vi "GetHeader2.vi"(8 "error in (no error)":errorcluster caption="에러 입력(에러 없음)", 11 "ABF1FIO 입력":refnum<class "ABF1FIO.lvclass">) -> (0 "error out":errorcluster caption="에러 출력", 1 "Header":T1, 3 "ABF1FIO 출력":refnum<class "ABF1FIO.lvclass">)   [LabVIEW 2017, in "ABF1FIO.lvclass"]
uses:
  ABF1FIO.lvclass
  ABF1FIO.lvclass/ABF1FIO.ctl
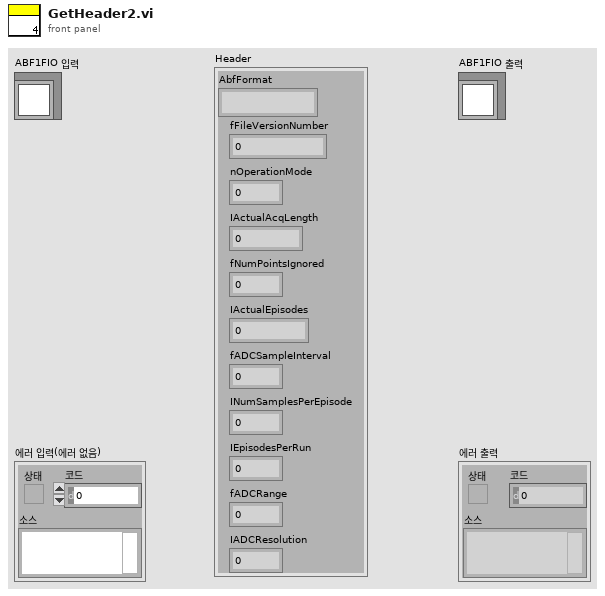
[diagram p1: front panel]
types:
  T1 = cluster{"AbfFormat":string, "fFileVersionNumber":sgl, "nOperationMode":i8, "IActualAcqLength":u32, "fNumPointsIgnored":i8, "IActualEpisodes":i32, "fADCSampleInterval":sgl, "INumSamplesPerEpisode":u32, "IEpisodesPerRun":u32, "fADCRange":sgl, "IADCResolution":u32}
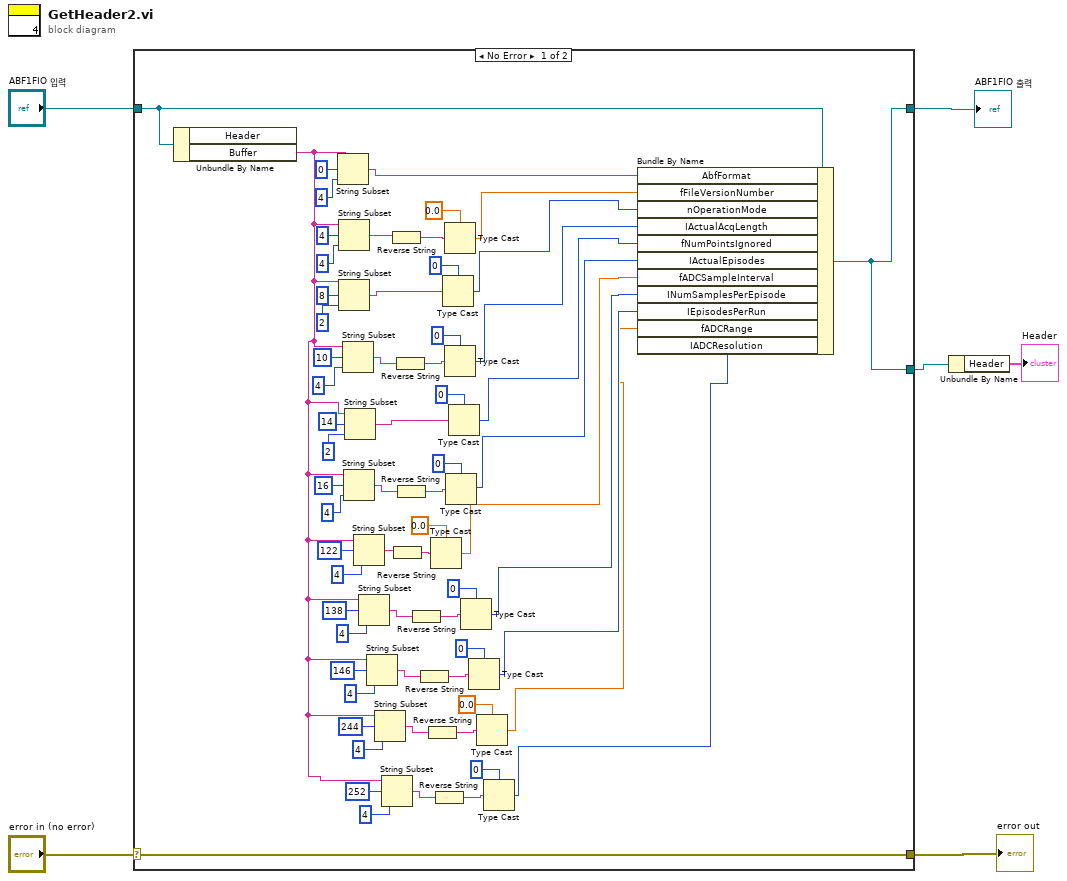
[diagram p0: block diagram]
diagram:
  n1 = case shown="No Error" "error in (no error)" {
    selector: "error in (no error)" -> [w71 w73]
    tunnel: [w71 w73] -> w5
    tunnel: [w7 w72] -> w3
    tunnel: "ABF1FIO 입력" -> [w19 w72]
    tunnel: [w7 _] -> w2
    frame No Error {
      n2 = Unbundle By Name(w19) -> ("Buffer"=w21:string)  [unwired: 1 out]
      n3 = String Subset(string=w21, offset (0)=0 ("오프셋(0)"), length (rest)=4 ("오프셋(0)")) -> (substring=w18:string)
      n4 = String Subset(string=w21, offset (0)=4 ("오프셋(0)"), length (rest)=4 ("오프셋(0)")) -> (substring=w64:string)
      n5 = String Subset(string=w21, offset (0)=8 ("오프셋(0)"), length (rest)=2 ("오프셋(0)")) -> (substring=w61:string)
      n6 = String Subset(string=w21, offset (0)=10 ("오프셋(0)"), length (rest)=4 ("길이(나머지)")) -> (substring=w57:string)
      n7 = String Subset(string=w21, offset (0)=16 ("오프셋(0)"), length (rest)=4 ("오프셋(0)")) -> (substring=w48:string)
      n8 = String Subset(string=w21, offset (0)=14 ("오프셋(0)"), length (rest)=2 ("오프셋(0)")) -> (substring=w51:string)
      n9 = String Subset(string=w21, offset (0)=122 ("오프셋(0)"), length (rest)=4 ("길이(나머지)")) -> (substring=w45:string)
      n10 = String Subset(string=w21, offset (0)=138 ("오프셋(0)"), length (rest)=4 ("길이(나머지)")) -> (substring=w39:string)
      n11 = String Subset(string=w21, offset (0)=146 ("오프셋(0)"), length (rest)=4 ("길이(나머지)")) -> (substring=w33:string)
      n12 = String Subset(string=w21, offset (0)=244 ("오프셋(0)"), length (rest)=4 ("길이(나머지)")) -> (substring=w28:string)
      n13 = String Subset(string=w21, offset (0)=252 ("오프셋(0)"), length (rest)=4 ("길이(나머지)")) -> (substring=w23:string)
      n14 = Reverse String(1:w64) -> (0:w66:string)
      n15 = Reverse String(1:w45) -> (0:w44:string)
      n16 = Reverse String(1:w57) -> (0:w55:string)
      n17 = Reverse String(1:w48) -> (0:w50:string)
      n18 = Reverse String(1:w39) -> (0:w38:string)
      n19 = Reverse String(1:w33) -> (0:w34:string)
      n20 = Reverse String(1:w28) -> (0:w27:string)
      n21 = Type Cast(type=sgl 0.0 ("오프셋(0)"), x=w44) -> (*(type *) &x=w12:sgl)
      n22 = Reverse String(1:w23) -> (0:w24:string)
      n23 = Type Cast(type=i8 0 ("오프셋(0)"), x=w61) -> (*(type *) &x=w16:i8)
      n24 = Type Cast(type=sgl 0.0 ("오프셋(0)"), x=w66) -> (*(type *) &x=w17:sgl)
      n25 = Type Cast(type=u32 0 ("오프셋(0)"), x=w55) -> (*(type *) &x=w15:u32)
      n26 = Type Cast(type=u32 0 ("오프셋(0)"), x=w50) -> (*(type *) &x=w13:u32)
      n27 = Type Cast(type=i8 0 ("오프셋(0)"), x=w51) -> (*(type *) &x=w14:i8)
      n28 = Type Cast(type=u32 0 ("오프셋(0)"), x=w38) -> (*(type *) &x=w11:u32)
      n29 = Type Cast(type=u32 0 ("오프셋(0)"), x=w34) -> (*(type *) &x=w10:u32)
      n30 = Type Cast(type=sgl 0.0 ("오프셋(0)"), x=w27) -> (*(type *) &x=w9:sgl)
      n31 = Type Cast(type=u32 0 ("오프셋(0)"), x=w24) -> (*(type *) &x=w8:u32)
      n32 = Bundle By Name(cluster=w19, "AbfFormat"=w18, "fFileVersionNumber"=w17, "nOperationMode"=w16, "IActualAcqLength"=w15, "fNumPointsIgnored"=w14, "IActualEpisodes"=w13, "fADCSampleInterval"=w12, "INumSamplesPerEpisode"=w11, "IEpisodesPerRun"=w10, "fADCRange"=w9, "IADCResolution"=w8) -> (w7:refnum<class "ABF1FIO.lvclass">)
    }
    frame Error {
    }
  }
  "error out" <- w5
  "ABF1FIO 출력" <- w3
  n33 = Unbundle By Name(w2) -> ("Header"=→"Header":T1)
